vi "OE1022D_Configure Ref Phase Channel A.vi"(0 "VISA resource name":refnum<visa-resource-name>, 1 "Reference Source":u8(ring) items=["External", "Internal", "Internal Sweep"], 2 "External Ref Trigger":u8(ring) items=["TTL Rising Edge", "Sine Zero Crossing"], 3 "Internal Frequency(Hz)":sgl=1000.0 format="%.3f", 4 "Phase  (degree)":sgl format="%.2f", 5 "error in (no error)":errorcluster, 6 "Sweep Mode":u8(ring) items=["Linear", "Log"], 7 "Linear Step Frequency(Hz)":sgl=1000.0 format="%.3f", 8 "Start Frequency(Hz)":sgl=1000.0 format="%.3f", 9 "Log Step Percent(%)":sgl=10.0 format="%.3f", 10 "Stop Frequency(Hz)":sgl=5000.0 format="%.3f", 11 "Sweep Run Mode":u8(ring) items=["Stop", "Single", "Loop"], 12 "Step Time(ms)":sgl=1000.0 min=1 max=100000) -> (14 "VISA resource name out":refnum<visa-resource-name>, 19 "error out":errorcluster)   [LabVIEW 2014]
doc: "Configures the reference source and the internal oscillator."
panel:
  out "结果字符串":string
  # "Signal Generator"
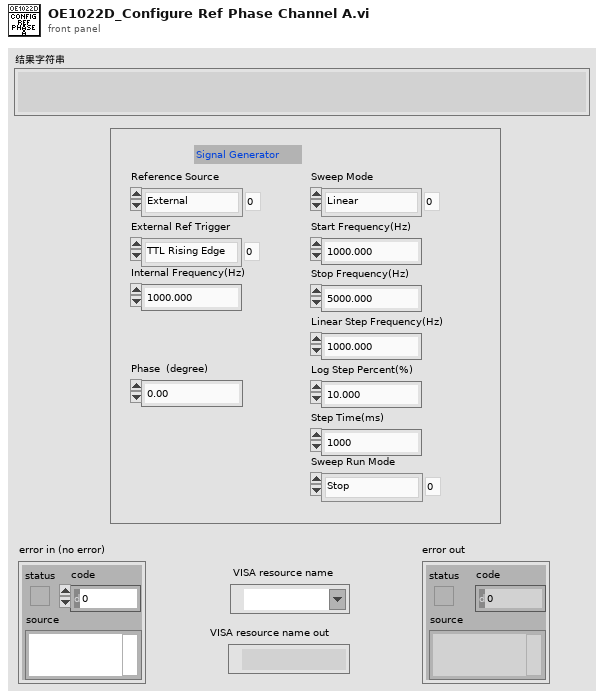
[diagram p1: front panel]
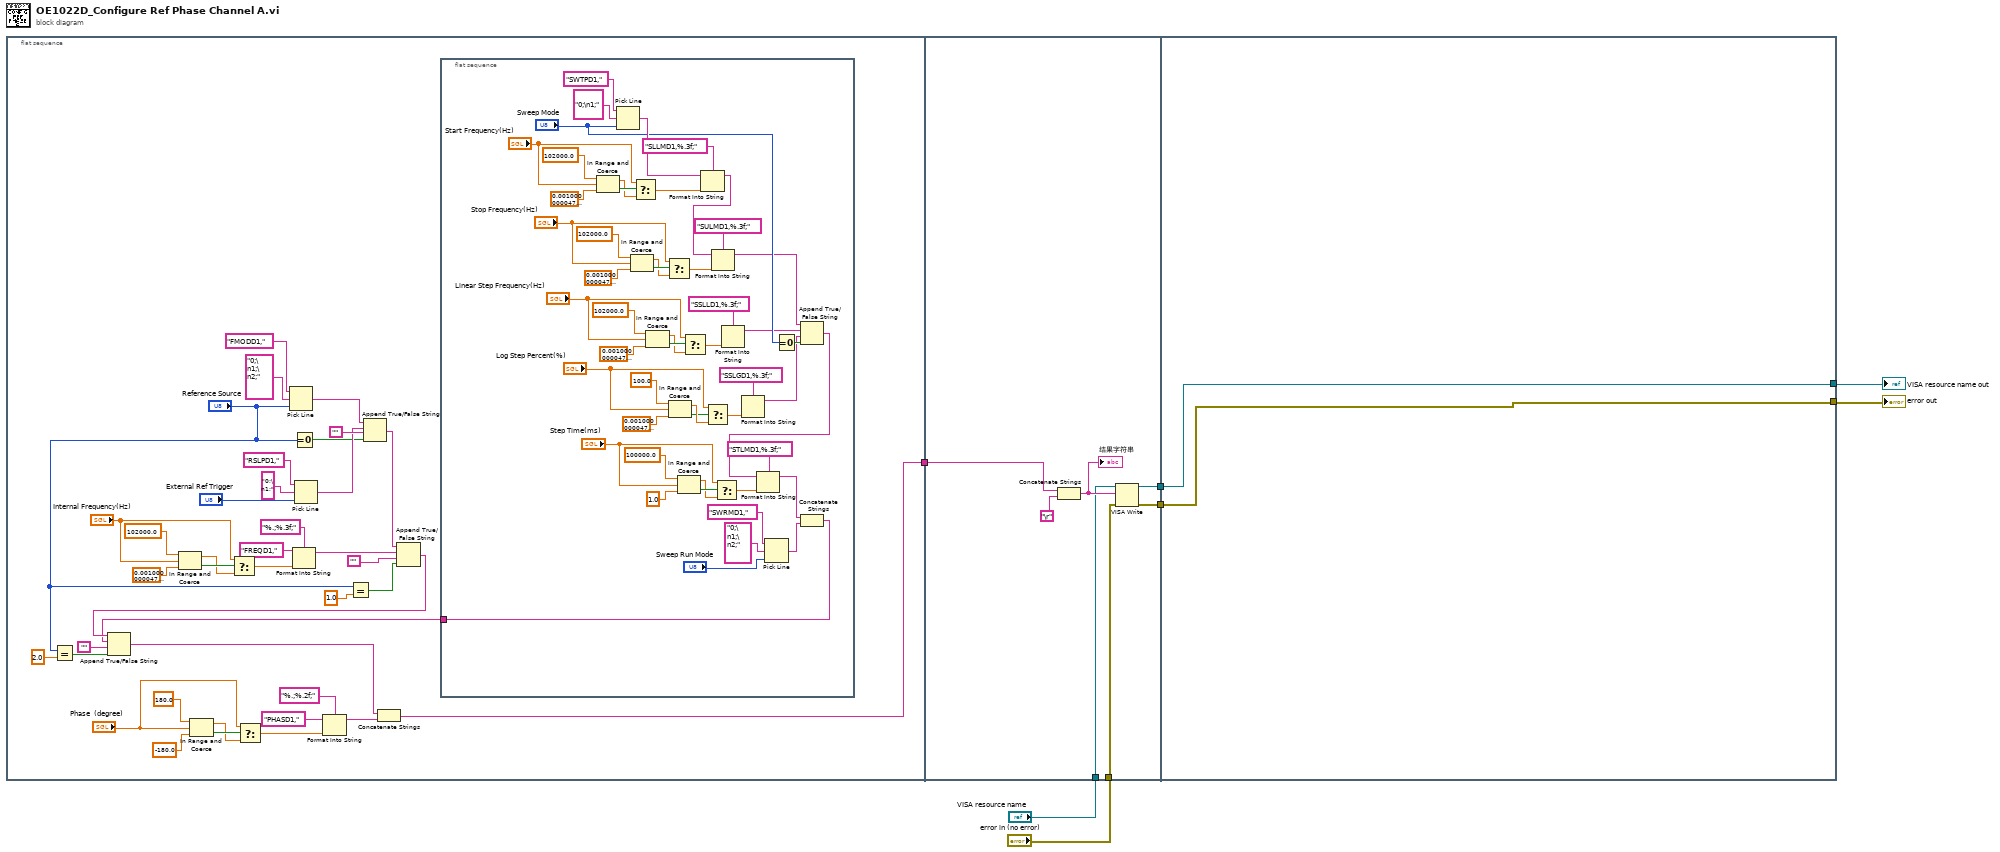
[diagram p0: block diagram]
diagram:
  n1 = flat-sequence {
    tunnel: [w9] -> w5
    tunnel: w5 -> [w102]
    tunnel: "VISA resource name" -> [w101]
    tunnel: "error in (no error)" -> [w100]
    tunnel: [w99] -> w4
    tunnel: [w98] -> w3
    tunnel: [w106] -> w7
    tunnel: [w105] -> w6
    tunnel: w4 -> [w106]
    tunnel: w3 -> [w105]
    frame #0 {
      n2 = Equal?(x="Reference Source", y=2.0) -> (x = y?=w18:bool)
      n3 = In Range and Coerce(upper limit=sgl 102000.0 ("上限"), x="Internal Frequency(Hz)", lower limit=sgl 0.001 ("下限")) -> (coerced(x)=w20:sgl, In Range?=w24:bool)
      n4 = In Range and Coerce(upper limit=sgl 180.0 ("上限"), x="Phase  (degree)", lower limit=sgl -180.0 ("下限")) -> (coerced(x)=w30:sgl, In Range?=w32:bool)
      n5 = Select(t="Internal Frequency(Hz)", s=w24, f=w20) -> (s? t:f=w45:sgl)
      n6 = Select(t="Phase  (degree)", s=w32, f=w30) -> (s? t:f=w27:sgl)
      n7 = Pick Line(string ("")="FMODD1,", multi-line string="0;\n1;\n2;", line index="Reference Source") -> (output string=w29:string)
      n8 = Format Into String(format string="%.;%.3f;", initial string="FREQD1,", w45) -> (resulting string=w14:string)  [unwired: 1 in, 1 out]
      n9 = Equal To 0?(x="Reference Source") -> (x = 0?=w35:bool)
      n10 = Pick Line(string ("")="RSLPD1,", multi-line string="0;\n1;", line index="External Ref Trigger") -> (output string=w37:string)
      n11 = Format Into String(format string="%.;%.2f;" ("格式字符串"), initial string="PHASD1,", w27) -> (resulting string=w25:string)  [unwired: 1 in, 1 out]
      n12 = Equal?(x="Reference Source", y=1.0) -> (x = y?=w10:bool)
      n13 = Append True/False String(1:w35, 2:"" ("false string"), 3:w37, 4:w29) -> (0:w36:string)
      n14 = Append True/False String(1:w10, 2:"" ("false string"), 3:w14, 4:w36) -> (0:w17:string)
      n15 = Append True/False String(1:w18, 2:"", 3:w15, 4:w17) -> (0:w8:string)
      n16 = Concatenate Strings(w8, w25) -> (w9:string)
      n17 = flat-sequence {
        tunnel: [w53] -> w15
        frame #0 {
          n18 = In Range and Coerce(upper limit=sgl 102000.0 ("上限"), x="Start Frequency(Hz)", lower limit=sgl 0.001 ("下限")) -> (coerced(x)=w89:sgl, In Range?=w93:bool)
          n19 = Pick Line(string ("")="SWTPD1,", multi-line string="0;\n1;", line index="Sweep Mode") -> (output string=w57:string)
          n20 = In Range and Coerce(upper limit=sgl 102000.0 ("上限"), x="Stop Frequency(Hz)", lower limit=sgl 0.001 ("下限")) -> (coerced(x)=w83:sgl, In Range?=w86:bool)
          n21 = Select(t="Start Frequency(Hz)", s=w93, f=w89) -> (s? t:f=w95:sgl)
          n22 = In Range and Coerce(upper limit=sgl 102000.0 ("上限"), x="Linear Step Frequency(Hz)", lower limit=sgl 0.001 ("下限")) -> (coerced(x)=w76:sgl, In Range?=w79:bool)
          n23 = Select(t="Stop Frequency(Hz)", s=w86, f=w83) -> (s? t:f=w88:sgl)
          n24 = In Range and Coerce(upper limit=sgl 100.0 ("上限"), x="Log Step Percent(%)", lower limit=sgl 0.001 ("下限")) -> (coerced(x)=w74:sgl, In Range?=w71:bool)
          n25 = In Range and Coerce(upper limit=sgl 100000.0 ("上限"), x="Step Time(ms)", lower limit=sgl 1.0 ("下限")) -> (coerced(x)=w62:sgl, In Range?=w65:bool)
          n26 = Select(t="Linear Step Frequency(Hz)", s=w79, f=w76) -> (s? t:f=w81:sgl)
          n27 = Format Into String(format string="SLLMD1,%.3f;", initial string=w57, w95) -> (resulting string=w56:string)  [unwired: 1 in, 1 out]
          n28 = Select(t="Log Step Percent(%)", s=w71, f=w74) -> (s? t:f=w69:sgl)
          n29 = Format Into String(format string="SULMD1,%.3f;", initial string=w56, w88) -> (resulting string=w48:string)  [unwired: 1 in, 1 out]
          n30 = Select(t="Step Time(ms)", s=w65, f=w62) -> (s? t:f=w67:sgl)
          n31 = Format Into String(format string="SSLLD1,%.3f;", w81) -> (resulting string=w50:string)  [unwired: 2 in, 1 out]
          n32 = Format Into String(format string="SSLGD1,%.3f;", w69) -> (resulting string=w49:string)  [unwired: 2 in, 1 out]
          n33 = Pick Line(string ("")="SWRMD1,", multi-line string="0;\n1;\n2;", line index="Sweep Run Mode") -> (output string=w55:string)
          n34 = Equal To 0?(x="Sweep Mode") -> (x = 0?=w52:bool)
          n35 = Append True/False String(1:w52, 2:w49, 3:w50, 4:w48) -> (0:w47:string)
          n36 = Format Into String(format string="STLMD1,%.3f;", initial string=w47, w67) -> (resulting string=w54:string)  [unwired: 1 in, 1 out]
          n37 = Concatenate Strings(w54, w55) -> (w53:string)
        }
      }
    }
    frame #1 {
      n38 = Concatenate Strings(w102, "\r") -> (w103:string)
      "结果字符串" <- w103
      n39 = VISA Write(VISA resource name=w101, write buffer=w103, error in (no error)=w100) -> (VISA resource name out=w99:refnum<visa-resource-name>, error out=w98:errorcluster)  [unwired: 1 out]
    }
    frame #2 {
    }
  }
  "error out" <- w6
  "VISA resource name out" <- w7
